vi "read_machine_parameters_mt_connect_1(SubVI).vi"(9 "URL 2":string="http://amrcadp:5000/current/", 11 "error in (no error) 3":errorcluster) -> (0 "error out 3":errorcluster, 2 "Machine Data":T1)   [LabVIEW 2014]
uses:
  <vilib>/addons/internet/NI_InternetTK_Core_VIs.lvlib
panel:
  out "concatenated string":string
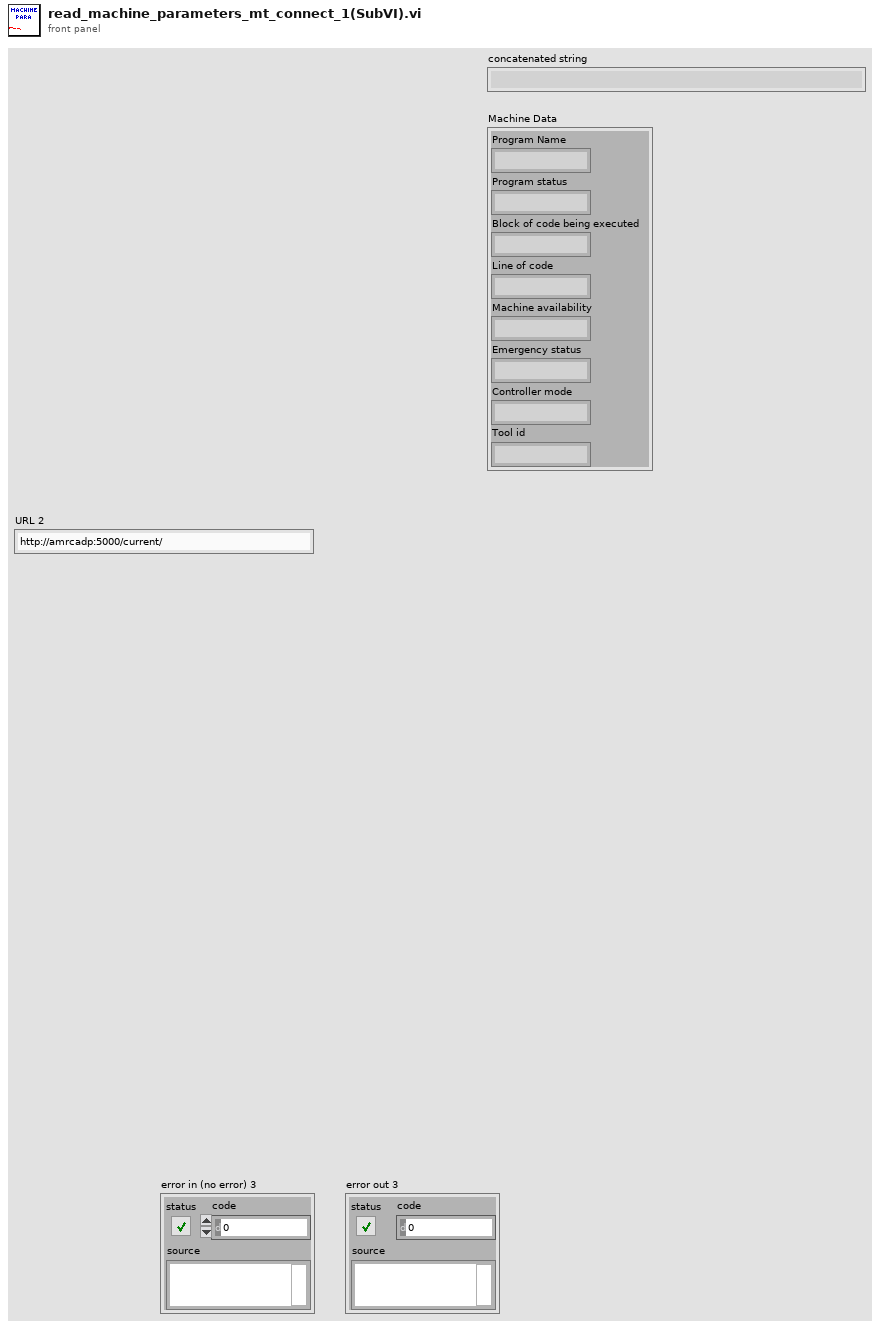
[diagram p1: front panel]
types:
  T1 = cluster{"Program Name":string, "Program status":string, "Block of code being executed":string, "Line of code":string, "Machine availability":string, "Emergency status":string, "Controller mode":string, "Tool id":string}
  T2 = cluster{"Result XML":string, "Result XML":string, "Result XML":string, "Result XML":string, "Result XML":string, "Result XML":string, "Result XML":string, "Result XML":string}
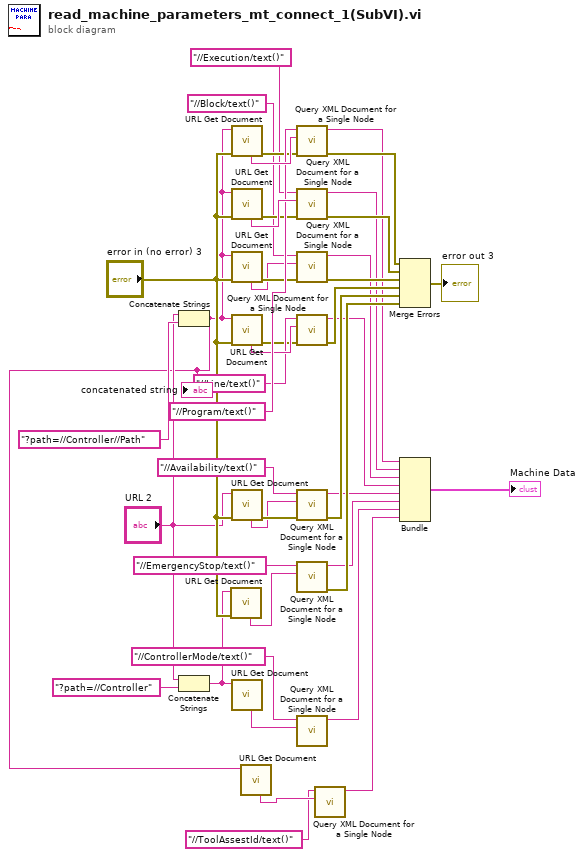
[diagram p0: block diagram]
diagram:
  n1 = Concatenate Strings("URL 2", "?path=//Controller//Path" ("string")) -> (w2:string)
  "concatenated string" <- w2
  n2 = Concatenate Strings("URL 2", "?path=//Controller" ("string")) -> (w21:string)
  n3 = call <vilib>:"URL Get Document.vi"("error in (no error)"="error in (no error) 3", "URL"=w21) -> ("content"=w29:string)  [unwired: 5 in, 4 out]
  n4 = call <vilib>:"URL Get Document.vi"("error in (no error)"="error in (no error) 3", "URL"=w2) -> ("error out"=w40:errorcluster, "content"=w42:string)  [unwired: 5 in, 3 out]
  n5 = call <vilib>:"URL Get Document.vi"("error in (no error)"="error in (no error) 3", "URL"=w2) -> ("error out"=w39:errorcluster, "content"=w43:string)  [unwired: 5 in, 3 out]
  n6 = call <vilib>:"URL Get Document.vi"("error in (no error)"="error in (no error) 3", "URL"=w2) -> ("error out"=w38:errorcluster, "content"=w36:string)  [unwired: 5 in, 3 out]
  n7 = call <vilib>:"URL Get Document.vi"("error in (no error)"="error in (no error) 3", "URL"=w2) -> ("error out"=w33:errorcluster, "content"=w35:string)  [unwired: 5 in, 3 out]
  n8 = call <vilib>:"URL Get Document.vi"("error in (no error)"="error in (no error) 3", "URL"="URL 2") -> ("error out"=w32:errorcluster, "content"=w30:string)  [unwired: 5 in, 3 out]
  n9 = call <vilib>:"URL Get Document.vi"("URL"=w21) -> ("content"=w26:string)  [unwired: 6 in, 4 out]
  n10 = call <vilib>:"URL Get Document.vi"("URL"=w2) -> ("content"=w11:string)  [unwired: 6 in, 4 out]
  n11 = call "Query XML Document for a Single Node.vi"("error in (no error)"=w40, "XML document"=w42, "XPath expression"="//Program/text()") -> ("error out"=w20:errorcluster, "Result XML"=w9:string)  [unwired: 6 in, 1 out]
  n12 = call "Query XML Document for a Single Node.vi"("error in (no error)"=w39, "XML document"=w43, "XPath expression"="//Execution/text()") -> ("error out"=w19:errorcluster, "Result XML"=w8:string)  [unwired: 6 in, 1 out]
  n13 = call "Query XML Document for a Single Node.vi"("error in (no error)"=w38, "XML document"=w36, "XPath expression"="//Block/text()") -> ("error out"=w18:errorcluster, "Result XML"=w13:string)  [unwired: 6 in, 1 out]
  n14 = call "Query XML Document for a Single Node.vi"("error in (no error)"=w33, "XML document"=w35, "XPath expression"="//Line/text()") -> ("error out"=w17:errorcluster, "Result XML"=w7:string)  [unwired: 6 in, 1 out]
  n15 = call "Query XML Document for a Single Node.vi"("error in (no error)"=w32, "XML document"=w30, "XPath expression"="//Availability/text()") -> ("error out"=w16:errorcluster, "Result XML"=w12:string)  [unwired: 6 in, 1 out]
  n16 = call "Query XML Document for a Single Node.vi"("XML document"=w29, "XPath expression"="//EmergencyStop/text()") -> ("error out"=w15:errorcluster, "Result XML"=w6:string)  [unwired: 7 in, 1 out]
  n17 = call "Query XML Document for a Single Node.vi"("XML document"=w26, "XPath expression"="//ControllerMode/text()") -> ("Result XML"=w5:string)  [unwired: 7 in, 2 out]
  n18 = call "Query XML Document for a Single Node.vi"("XML document"=w11, "XPath expression"="//ToolAssestId/text()") -> ("Result XML"=w4:string)  [unwired: 7 in, 2 out]
  n19 = Merge Errors(w20, w19, w18, w17, w16, w15) -> (→"error out 3":errorcluster)
  n20 = Bundle("Result XML"=w9, "Result XML"=w8, "Result XML"=w13, "Result XML"=w7, "Result XML"=w12, "Result XML"=w6, "Result XML"=w5, "Result XML"=w4) -> (→"Machine Data":T2)  [unwired: 1 in]
